vi "final_gauss_fit.vi"(4 "Input X":sgl[](array[numeric]) format="%.2f", 7 "max iteration":i32=300, 8 "Input Y":sgl[](array[numeric]) format="%.2f") -> (0 "Best Fit":dbl[](array[numeric]) format="%.2f", 1 "Fit (Y)":dbl[](array[numeric]) format="%.2f", 2 "Iterations":i32, 3 "Fit Results":T1 {"FWHM" format="%.3f"; "Offset" format="%.3f"; "Amplitude" format="%.3f"; "Position" format="%.3f"}, 5 "Positions (X)":dbl[](array[numeric]) format="%.2f", 6 "Data (Y)":dbl[](array[numeric]) format="%.2f")   [LabVIEW 2013]
uses:
  <vilib>/Analysis/NI_AALPro.lvlib
panel:
  out "log(sum_y atoms) -log(sum_y backgnd):\n X density distribution":cluster{"Input X":sgl[], "Input Y":sgl[]}(graph)
  out "Initial guess":dbl[](array[numeric]) format="%.2f"
  # "The Initial amplitude guess is the largest value in file. So the Guassian must\nbe postive. Initial background guess is zero."
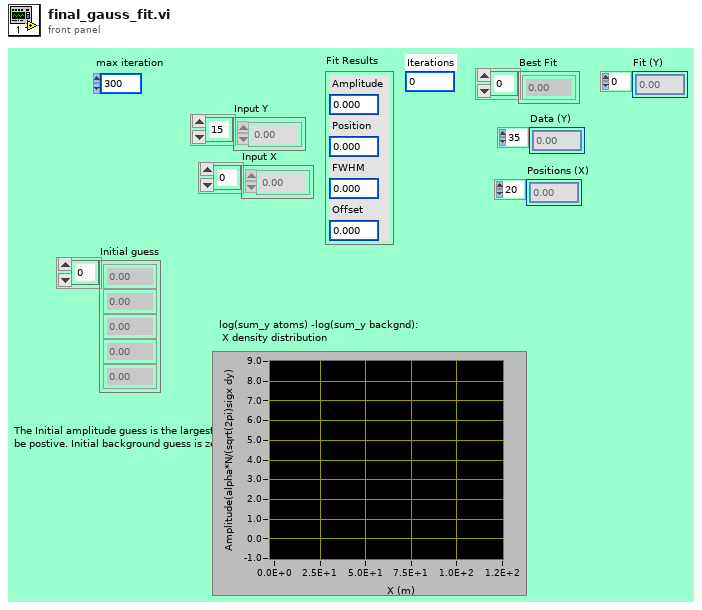
[diagram p1: front panel]
types:
  T1 = cluster{"Amplitude":dbl, "Position":dbl, "FWHM":dbl, "Offset":dbl}
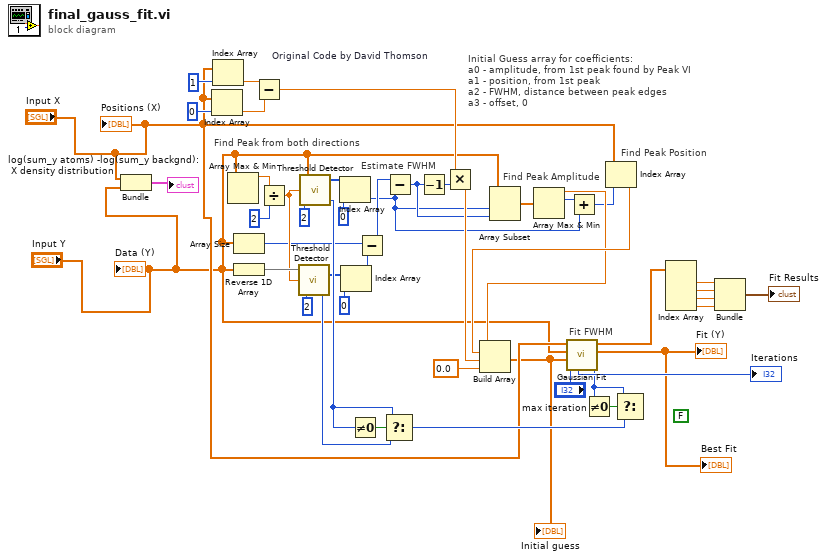
[diagram p0: block diagram]
diagram:
  (unwired) FALSE ("Error (T)")
  # "Find Peak from both directions"
  # "Fit FWHM"
  # "Initial Guess array for coefficients:\na0 - amplitude, from 1st peak found by Peak VI\na1 - position, from 1st peak\na2 - FWHM, distance between peak edges\na3 - offset, 0"
  # "Find Peak Amplitude"
  # "Find Peak Position"
  # "Estimate FWHM"
  n1 = Bundle("Input X"="Input X", "Input Y"="Input Y") -> (→"log(sum_y atoms) -log(sum_y backgnd):\n X density distribution":cluster{"Input X":sgl[], "Input Y":sgl[]})  [unwired: 1 in]
  n2 = Index Array(array="Input X", index=0) -> (element=w33:sgl)
  n3 = Index Array "Original Code by David Thomson"(array="Input X", index=1) -> (element=w32:sgl)
  n4 = Array Max & Min(array="Input Y") -> (max value=w26:sgl)  [unwired: 3 out]
  n5 = Array Size(array="Input Y") -> (size(s)=w18:i32)
  n6 = Reverse 1D Array(array="Input Y") -> (reversed array=w23:sgl[])
  n7 = Subtract(x=w32, y=w33) -> (x-y=w34:sgl)
  n8 = Divide(x=w26, y=2) -> (x/y=w22:sgl)
  n9 = call <vilib>:"Threshold Detector.vi"("width"=2, "threshold"=w22, "X"=w23) -> ("error"=w37:i32, "Indices"=w19:i32[])  [unwired: 1 out]
  n10 = call <vilib>:"Threshold Detector.vi"("width"=2, "threshold"=w22, "X"="Input Y") -> ("error"=w36:i32, "Indices"=w27:i32[])  [unwired: 1 out]
  n11 = Index Array(array=w27, index=0) -> (element=w7:i32)
  n12 = Index Array(array=w19, index=0) -> (element=w17:i32)
  n13 = Not Equal To 0?(x=w36) -> (x != 0?=w35:bool)
  n14 = Subtract(x=w18, y=w17) -> (x-y=w14:i32)
  n15 = Select(t=w36, s=w35, f=w37) -> (s? t:f=w40:i32)
  n16 = Subtract(x=w14, y=w7) -> (x-y=w12:i32)
  n17 = Decrement(x=w12) -> (x-1=w13:i32)
  n18 = Multiply(x=w34, y=w13) -> (x*y=w15:sgl)
  n19 = Array Subset(array="Input Y", index=w7, length=w12) -> (w11:sgl[])
  n20 = Array Max & Min(array=w11) -> (max value=w10:sgl, max index (indices)=w8:i32)  [unwired: 2 out]
  n21 = Add(x=w8, y=w7) -> (x+y=w9:i32)
  n22 = Index Array(array="Input X", index=w9) -> (element=w16:sgl)
  n23 = Build Array(w10, w16, w15, 0.0) -> (w4:dbl[])
  "Initial guess" <- w4
  n24 = call "Gaussian Fit.VI"("max iteration"="max iteration", "Initial Guess Coefficients"=w4, "Y"="Input Y", "X"="Input X") -> ("error"=w39:i32, "Best Fit"=→"Fit (Y)" →"Best Fit":dbl[], "Best Fit Coefficients"=w2:dbl[], "Iterations"=→"Iterations":i32)  [unwired: 1 in, 2 out]
  n25 = Not Equal To 0?(x=w39) -> (x != 0?=w38:bool)
  n26 = Select(t=w39, s=w38, f=w40) -> ()  [unwired: 1 out]
  n27 = Index Array(array=w2) -> (element #1=w42:dbl, element #2=w43:dbl, element #3=w44:dbl, element #4=w45:dbl)  [unwired: 4 in]
  n28 = Bundle(w42, w43, w44, w45) -> (→"Fit Results":cluster{dbl, dbl, dbl, dbl})  [unwired: 1 in]
  "Data (Y)" <- "Input Y"
  "Positions (X)" <- "Input X"
